vi "getScore.vi"(8 "error in (no error)":errorcluster, 10 "call":i32, 11 "BingoBoard in":refnum<class "BingoBoard.lvclass">) -> (0 "error out":errorcluster, 2 "Score":i32, 3 "BingoBoard out":refnum<class "BingoBoard.lvclass">)   [LabVIEW 2017, in "BingoBoard.lvclass"]
uses:
  BingoBoard.lvclass
  BingoBoard.lvclass/BingoBoard.ctl
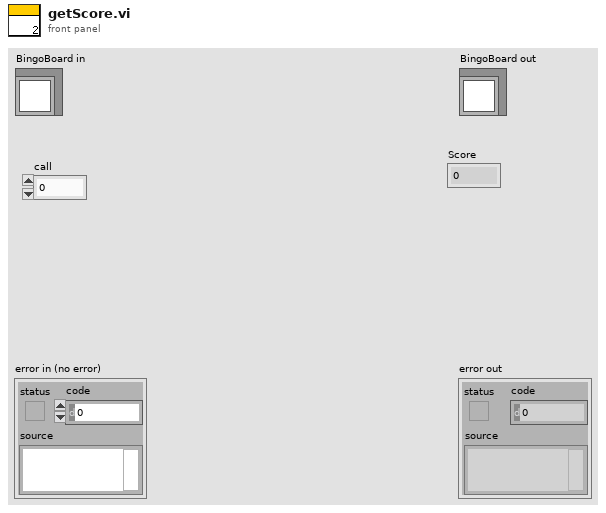
[diagram p1: front panel]
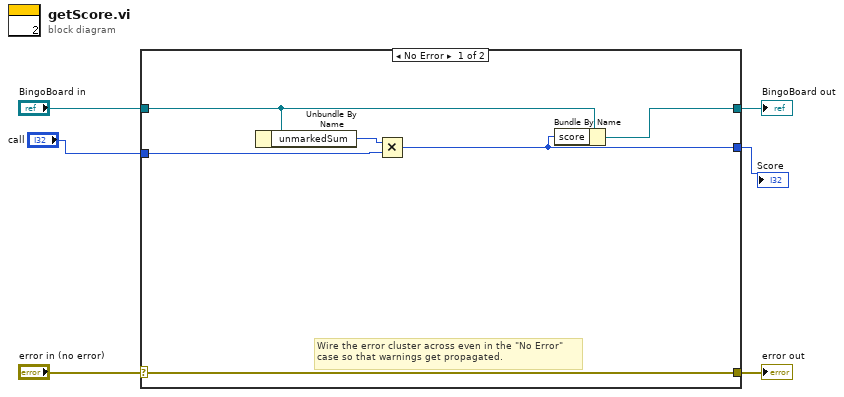
[diagram p0: block diagram]
diagram:
  n1 = case shown="No Error" "error in (no error)" {
    selector: "error in (no error)" -> [w12 w14]
    tunnel: [w12 w14] -> w5
    tunnel: [w8 w13] -> w3
    tunnel: "BingoBoard in" -> [w9 w13]
    tunnel: "call" -> [w10 _]
    tunnel: [w7 _] -> w1
    frame No Error {
      # "Wire the error cluster across even in the \"No Error\"\ncase so that warnings get propagated."
      n2 = Unbundle By Name(w9) -> ("unmarkedSum"=w11:i32)
      n3 = Multiply(x=w11, y=w10) -> (x*y=w7:i32)
      n4 = Bundle By Name(cluster=w9, "score"=w7) -> (w8:refnum<class "BingoBoard.lvclass">)
    }
    frame Error {
    }
  }
  "error out" <- w5
  "BingoBoard out" <- w3
  "Score" <- w1
